vi "Load-Save Color Lists.vi"(8 "error in (no error)":errorcluster, 10 "Load (F)/Save":bool, 11 "ini File Refnum in":T1) -> (0 "error out":errorcluster, 3 "ini File Refnum out":T1)   [LabVIEW 2019]
uses:
  <vilib>/Utility/config.llb/Config Data RefNum.ctl
  <vilib>/Utility/config.llb/NI_LVConfig.lvlib
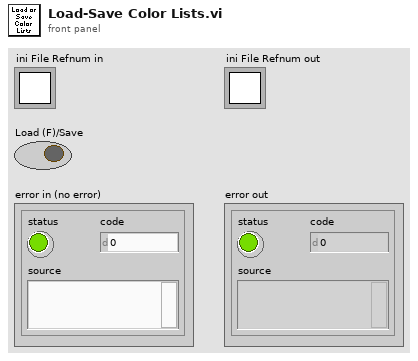
[diagram p1: front panel]
types:
  T1 = typedef "NI_LVConfig.lvlib/Config Data RefNum.ctl" = refnum<k1>
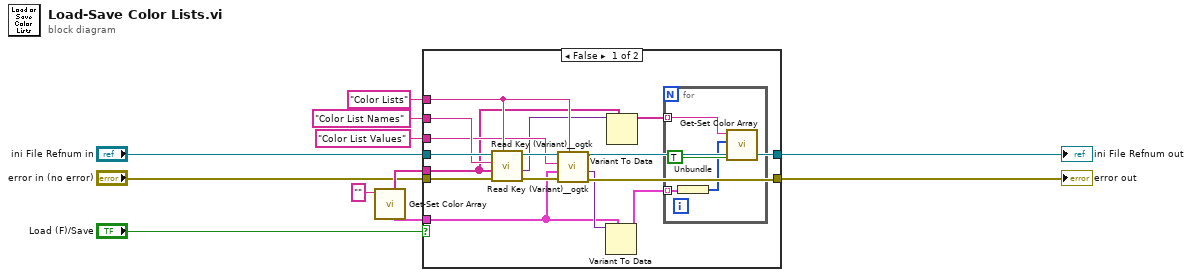
[diagram p0: block diagram]
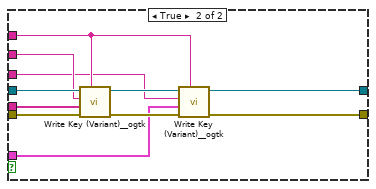
[diagram p2: hidden frame]
diagram:
  n1 = call "Get-Set Color Array.vi"("Color List Name"="") -> ("Color Arrays (out)"=w9:cluster{"Color Array":u32[]}[], "Color List Name (out)"=w10:string[])  [unwired: 5 in, 4 out]
  n2 = case shown="False" "Load (F)/Save" {
    tunnel: "ini File Refnum in" -> [w26 w41]
    tunnel: [w20 w38] -> w4
    tunnel: [w21 w37] -> w2
    tunnel: "error in (no error)" -> [w25 w31]
    tunnel: "Color Lists" ("section") -> [w19 w36]
    tunnel: "Color List Names" ("key (optional)") -> [w24 w35]
    tunnel: "Color List Values" ("key (optional)") -> [w18 w34]
    tunnel: w9 -> [w13 w33]
    tunnel: w10 -> [w15 w32]
    frame False {
      n3 = call <userlib>:"Read Key (Variant)__ogtk.vi"("section"=w19, "error in (no error)"=w25, "type"=w15, "key (optional)"=w24, "refnum"=w26) -> ("error out"=w22:errorcluster, "key-value"=w17:variant, "refnum out"=w23:T1)  [unwired: 3 in, 1 out]
      n4 = call <userlib>:"Read Key (Variant)__ogtk.vi"("section"=w19, "error in (no error)"=w22, "type"=w13, "key (optional)"=w18, "refnum"=w23) -> ("error out"=w21:errorcluster, "key-value"=w14:variant, "refnum out"=w20:T1)  [unwired: 3 in, 1 out]
      n5 = Variant To Data(type=w13, Variant=w14) -> (data=w12:cluster{"Color Array":u32[]}[])  [unwired: 1 in, 1 out]
      n6 = Variant To Data(type=w15, Variant=w17) -> (data=w16:string[])  [unwired: 1 in, 1 out]
      n7 = for {
        tunnel: w16 -> [w29] mode=indexing
        tunnel: w12 -> [w28] mode=indexing
        n8 = Unbundle(w28) -> ("Color Array"=w27:u32[])
        n9 = call "Get-Set Color Array.vi"("Get (F)/Set (T)"=TRUE, "Color Array (in)"=w27, "Color List Name"=w29) -> ()  [unwired: 3 in, 6 out]
      }
    }
    frame True {
      n10 = call <userlib>:"Write Key (Variant)__ogtk.vi"("section"=w36, "error in (no error)"=w31, "key-value"=w32, "key (optional)"=w35, "refnum"=w41) -> ("error out"=w39:errorcluster, "refnum out"=w40:T1)  [unwired: 5 in]
      n11 = call <userlib>:"Write Key (Variant)__ogtk.vi"("section"=w36, "error in (no error)"=w39, "key-value"=w33, "key (optional)"=w34, "refnum"=w40) -> ("error out"=w37:errorcluster, "refnum out"=w38:T1)  [unwired: 5 in]
    }
  }
  "ini File Refnum out" <- w4
  "error out" <- w2
